vi "Backpressure - drop-oldest.vi"(8 "error in (no error)":errorcluster) -> (0 "error out":errorcluster)   [LabVIEW 2026, in "Tests.lvlib"]
doc: "Update with test documentation"
uses:
  src/TypeDefs/Statement.ctl
  src/TypeDefs/Severity.ctl
  src/TypeDefs/DropPolicy.ctl
  <vilib>/addons/_JKI Toolkits/Caraya/classes/Assert/Assert True.vi
  <vilib>/addons/_JKI Toolkits/Caraya/classes/Assert/Assert Equal Value_Variant.vi
  <vilib>/addons/_JKI Toolkits/Caraya/classes/Assert/Assert False.vi
  Tests.lvlib
  <vilib>/addons/_JKI Toolkits/Caraya/classes/Test/Test.lvclass
  src/Lumberjack.lvlib
  <vilib>/addons/_JKI Toolkits/Caraya/classes/Assert/Assert.lvclass
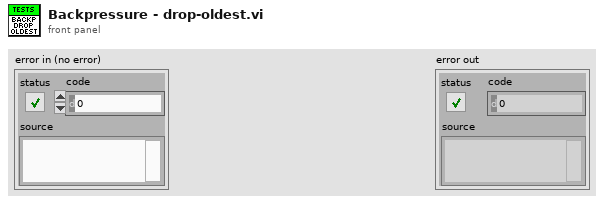
[diagram p1: front panel]
types:
  T1 = typedef "Lumberjack.lvlib/Severity.ctl" = enum16{"OFF", "FATAL", "ERROR", "WARN", "INFO", "DEBUG", "TRACE", "ALL"}
  T2 = typedef "Lumberjack.lvlib/DropPolicy.ctl" = enum16{"DropOldest", "DropNewest", "LevelAware"}
  T3 = typedef "Lumberjack.lvlib/Statement.ctl" = cluster{"timestamp":timestamp, "level":T1, "sourceTag":string, "originVI":string, "message":string}
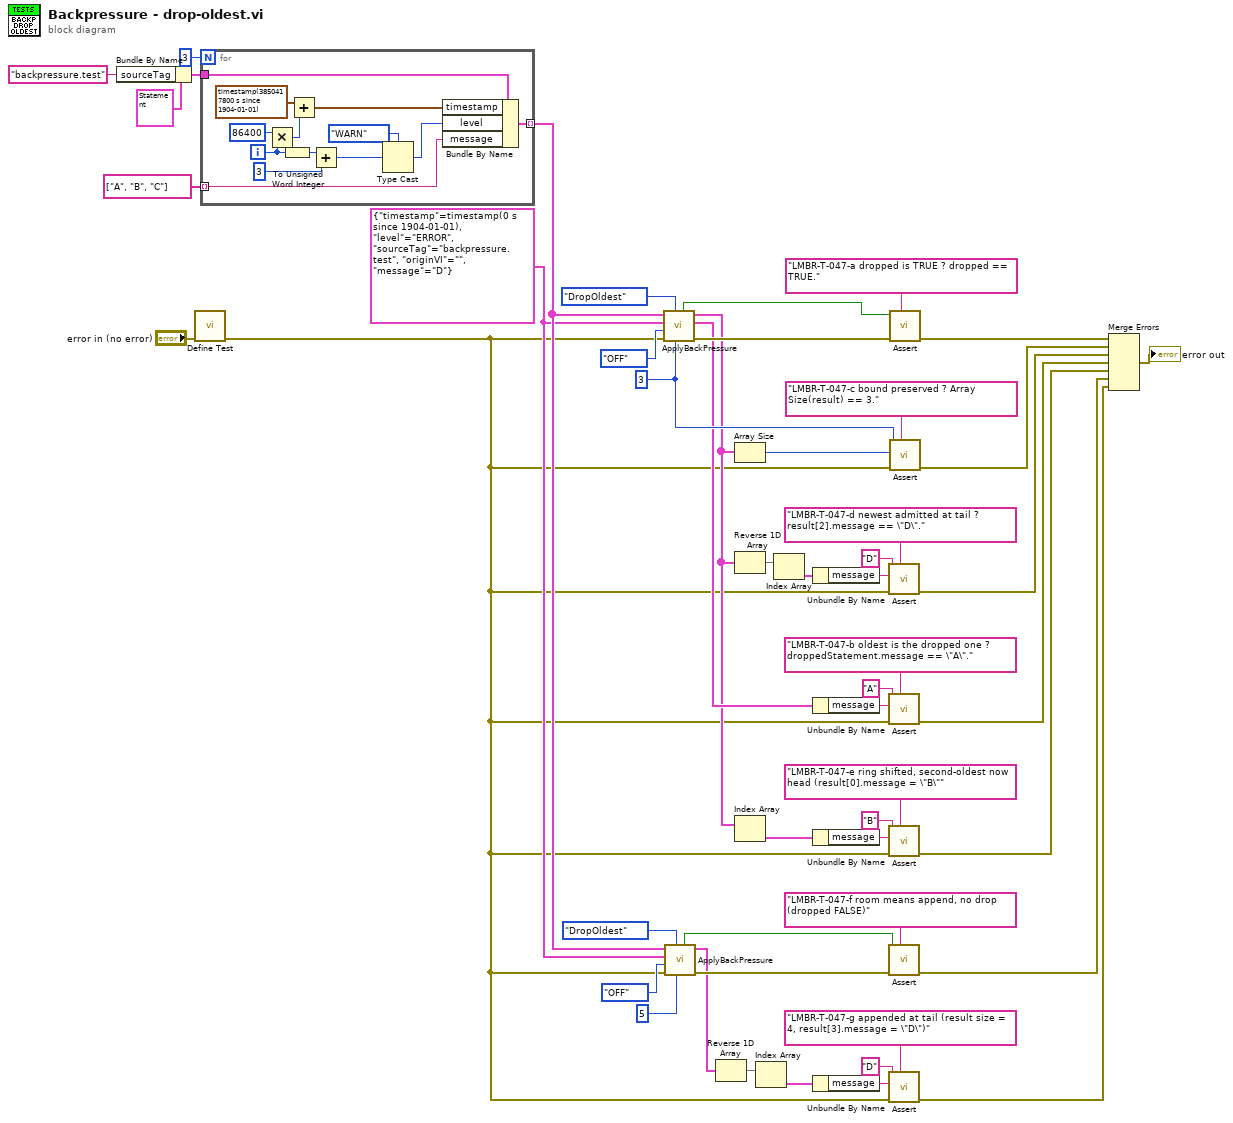
[diagram p0: block diagram]
diagram:
  w13 = T3 {"timestamp"=timestamp(0 s since 1904-01-01), "level"=enum."ERROR", "sourceTag"="backpressure.test", "originVI"="", "message"="D"} ("incoming")
  w39 = 3 ("queueBound")
  n1 = Bundle By Name(cluster=T3 {"timestamp"=timestamp(0 s since 1904-01-01), "level"=enum."INFO", "sourceTag"="", "originVI"="", "message"=""} ("Statement"), "sourceTag"="backpressure.test") -> (w47:T3)
  n2 = call <vilib>:"Define Test.vi"("error in (no error)"="error in (no error)") -> ("error out"=w5:errorcluster)  [unwired: 9 in, 1 out]
  n3 = for {
    N: 3 -> [_]
    tunnel: w47 -> [w61]
    tunnel: string[] ["A", "B", "C"] -> [w53] mode=indexing
    tunnel: [w52] -> w14 mode=indexing
    i -> [w59]
    n4 = Multiply(x=86400, y=w59) -> (x*y=w63:i32)
    n5 = To Unsigned Word Integer(number=w59) -> (unsigned 16bit integer=w58:u16)
    n6 = Add(x=timestamp(3850417800 s since 1904-01-01), y=w63) -> (x+y=w60:timestamp)
    n7 = Add(x=w58, y=u16 3) -> (x+y=w55:u16)
    n8 = Type Cast(type=Severity."WARN" ("level"), x=w55) -> (*(type *) &x=w54:T1)
    n9 = Bundle By Name(cluster=w61, "timestamp"=w60, "level"=w54, "message"=w53) -> (w52:T3)
  }
  n10 = call "ApplyBackPressure.vi"("queueBound"=w39, "DropPolicy"=DropPolicy."DropOldest", "error in (no error)"=w5, "worstSeverityIn"=Severity."OFF", "incoming"=w13, "pending"=w14) -> ("error out"=w42:errorcluster, "droppedStatement"=w34:T3, "result"=w25:T3[], "dropped"=w41:bool)  [unwired: 1 in, 1 out]
  n11 = call "ApplyBackPressure.vi"("queueBound"=5, "DropPolicy"=DropPolicy."DropOldest", "error in (no error)"=w5, "worstSeverityIn"=Severity."OFF", "incoming"=w13, "pending"=w14) -> ("error out"=w11:errorcluster, "result"=w2:T3[], "dropped"=w10:bool)  [unwired: 1 in, 2 out]
  n12 = Reverse 1D Array(array=w2) -> (reversed array=w1:T3[])
  n13 = Array Size(array=w25) -> (size(s)=w38:i32)
  n14 = Reverse 1D Array(array=w25) -> (reversed array=w30:T3[])
  n15 = Index Array(array=w25) -> (element=w21:T3)  [unwired: 1 in]
  n16 = Index Array(array=w1) -> (element=w6:T3)  [unwired: 1 in]
  n17 = Index Array(array=w30) -> (element=w26:T3)  [unwired: 1 in]
  n18 = Unbundle By Name(w26) -> ("message"=w27:string)
  n19 = Unbundle By Name(w34) -> ("message"=w33:string)
  n20 = Unbundle By Name(w21) -> ("message"=w22:string)
  n21 = Unbundle By Name(w6) -> ("message"=w7:string)
  n22 = call-poly <vilib>:"Assert.vi"("Label"="LMBR-T-047-d newest admitted at tail ? result[2].message == \"D\"." ("sourceTag"), "error in (no error)"=w5, "Actual"=w27, "Expected"="D") -> ("error out"=w20:errorcluster)  [unwired: 6 in, 1 out]
  n23 = call-poly <vilib>:"Assert.vi"("Label"="LMBR-T-047-b oldest is the dropped one ? droppedStatement.message == \"A\"." ("sourceTag"), "error in (no error)"=w5, "Actual"=w33, "Expected"="A") -> ("error out"=w19:errorcluster)  [unwired: 6 in, 1 out]
  n24 = call-poly <vilib>:"Assert.vi"("Label"="LMBR-T-047-e ring shifted, second-oldest now head (result[0].message = \"B\"" ("sourceTag"), "error in (no error)"=w5, "Actual"=w22, "Expected"="B") -> ("error out"=w18:errorcluster)  [unwired: 6 in, 1 out]
  n25 = call-poly <vilib>:"Assert.vi"("Label"="LMBR-T-047-f room means append, no drop (dropped FALSE)" ("sourceTag"), "error in (no error)"=w11, "False?"=w10) -> ("error out"=w4:errorcluster)  [unwired: 7 in, 1 out]
  n26 = call-poly <vilib>:"Assert.vi"("Label"="LMBR-T-047-g appended at tail (result size = 4, result[3].message = \"D\")" ("sourceTag"), "error in (no error)"=w5, "Actual"=w7, "Expected"="D") -> ("error out"=w3:errorcluster)  [unwired: 6 in, 1 out]
  n27 = call-poly <vilib>:"Assert.vi"("Label"="LMBR-T-047-a dropped is TRUE ? dropped == TRUE." ("sourceTag"), "error in (no error)"=w42, "True?"=w41) -> ("error out"=w32:errorcluster)  [unwired: 7 in, 1 out]
  n28 = call-poly <vilib>:"Assert.vi"("Label"="LMBR-T-047-c bound preserved ? Array Size(result) == 3." ("sourceTag"), "error in (no error)"=w5, "Actual"=w38, "Expected"=w39) -> ("error out"=w31:errorcluster)  [unwired: 6 in, 1 out]
  n29 = Merge Errors(w32, w31, w20, w19, w18, w4, w3) -> (→"error out":errorcluster)
